vi "SV Statistical Level.vi"   [LabVIEW 2017]
doc: "Use this VI to return <B>L_N</B> levels where L_N is the level which N % of the values exceed. For example, L50 represents the median, where 50 % of the values are greater than L_N and 50 % are lower. L90 is commonly used as a noise baseline, as 90 % of the values exceed L_N. L10 is commonly used as a measure of peak levels because it corresponds to the highest 10 % of levels."
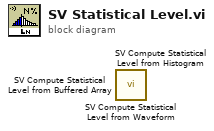
[diagram p0: block diagram]
diagram:
  n1 = call <vilib>:"SV Compute Statistical Level from Waveform.vi"() -> ()  [unwired: 14 in, 2 out]
  n2 = call <vilib>:"SV Compute Statistical Level from Histogram.vi"() -> ()  [unwired: 14 in, 2 out]
  n3 = call <vilib>:"SV Compute Statistical Level from Buffered Array.vi"() -> ()  [unwired: 14 in, 2 out]
